vi "Read Recurse.vi"(7 "Append Name (T)":bool=TRUE, 8 "Error In":errorcluster, 9 "Variant DB":variant, 10 "Name":string, 11 "Variant":variant) -> (0 "Error Out":errorcluster, 2 "String":string)   [LabVIEW 2017, in "Configit.lvlib"]
uses:
  Configit.lvlib
  <vilib>/Waveform/DTblOps.llb/DTbl Empty Digital.vi
  <vilib>/Waveform/DWDTOps.llb/DWDT Empty Digital.vi
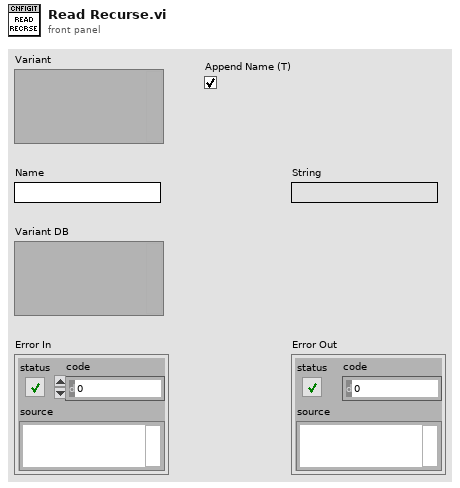
[diagram p1: front panel]
types:
  T1 = typedef "VariantType.lvlib/Type.ctl" = enum8{"Invalid Type", "Void", "I8", "I16", "I32", "I64", "U8", "U16", "U32", "U64", "Single Float", "Double Float", "Extended Float", "Single Complex", "Double Complex", "Extended Complex", "Enum U8", "Enum U16", "Enum U32", "Enum U64", "Single Float With Unit", "Double Float With Unit", "Extended Float With Unit", "Single Complex with Unit", "Double Complex with Unit", "Extended Complex with Unit", "Boolean", "String", "Path", "Picture", "Tag", "Array", "Cluster", "Variant", "LV Variant", "Waveform", "Timestamp", "Digital Waveform", "Digital Data", "ExpressData", "Refnum", "External Data", "VI", "Poly VI", "LabVIEW Class Instance", "Fixed Point"}
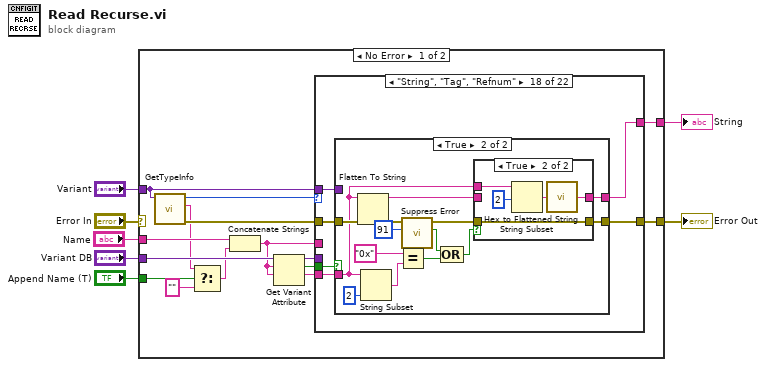
[diagram p0: block diagram]
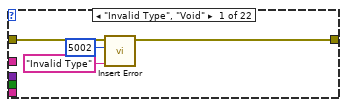
[diagram p2: hidden frame]
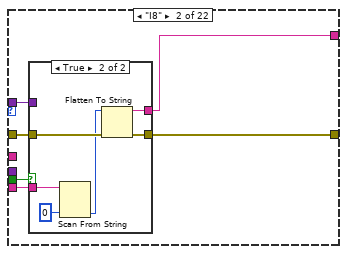
[diagram p3: hidden frame]
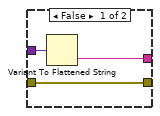
[diagram p4: hidden frame]
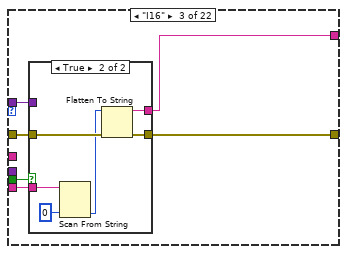
[diagram p5: hidden frame]
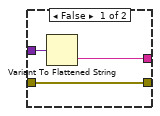
[diagram p6: hidden frame]
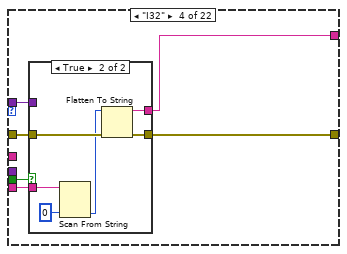
[diagram p7: hidden frame]
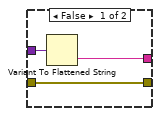
[diagram p8: hidden frame]
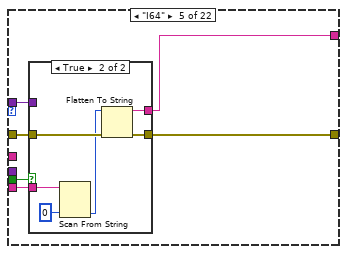
[diagram p9: hidden frame]
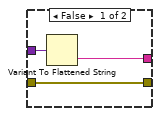
[diagram p10: hidden frame]
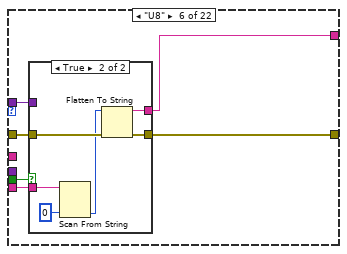
[diagram p11: hidden frame]
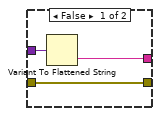
[diagram p12: hidden frame]
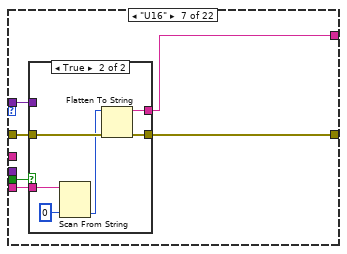
[diagram p13: hidden frame]
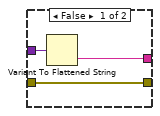
[diagram p14: hidden frame]
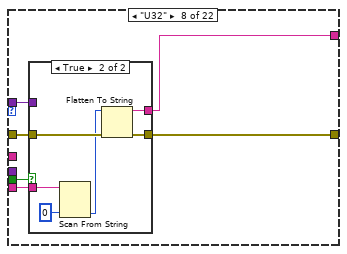
[diagram p15: hidden frame]
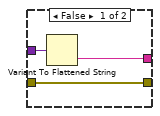
[diagram p16: hidden frame]
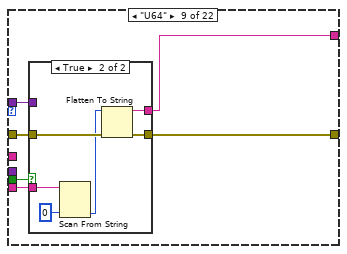
[diagram p17: hidden frame]
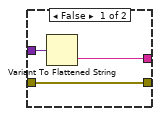
[diagram p18: hidden frame]
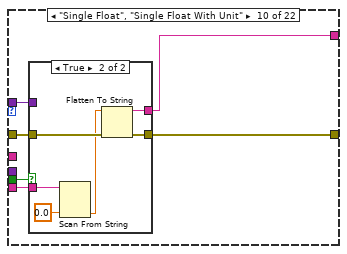
[diagram p19: hidden frame]
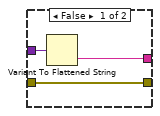
[diagram p20: hidden frame]
diagram:
  n1 = case shown="No Error" "Error In" {
    selector: "Error In" -> [_ w387]
    tunnel: "Variant" -> [w21 _]
    tunnel: "Name" -> [w18 _]
    tunnel: [w19 w387] -> w4
    tunnel: "Variant DB" -> [w17 _]
    tunnel: [w12 _] -> w2
    tunnel: "Append Name (T)" -> [w11 _]
    frame No Error {
      n2 = call "GetTypeInfo.vi"("Variant"=w21) -> ("Error Out"=w20:errorcluster, "Name"=w10:string, "Type Enum"=w22:T1)  [unwired: 7 in, 1 out]
      n3 = Select(t=w10, s=w11, f="") -> (s? t:f=w9:string)
      n4 = Concatenate Strings(w18, w9) -> (w13:string)
      n5 = Get Variant Attribute(Variant=w17, name=w13, default value (empty Variant)=w13) -> (duplicate Variant=w14:variant, found=w16:bool, value=w15:string)  [unwired: 1 in, 1 out]
      n6 = case shown="\"String\", \"Tag\", \"Refnum\"" w22 {
        tunnel: w21 -> [_ w28 w43 w58 w73 w88 w103 w118 w133 w148 w163 w178 w193 w214 w235 w256 w277 w293 w323 w339 w364 w374]
        tunnel: w20 -> [w26 w31 w46 w61 w76 w91 w106 w121 w136 w151 w166 w181 w196 w217 w238 w259 w280 w296 w326 w342 w365 w377]
        tunnel: [w23 w29 w44 w59 w74 w89 w104 w119 w134 w149 w164 w179 w194 w215 w236 w257 w278 w294 w324 w340 w354 w375] -> w19
        tunnel: w16 -> [_ w30 w45 w60 w75 w90 w105 w120 w135 w150 w165 w180 w195 w216 w237 w258 w279 w295 w325 w341 _ w376]
        tunnel: w15 -> [_ w32 w47 w62 w77 w92 w107 w122 w137 w152 w167 w182 w197 w218 w239 w260 w281 w297 w327 w343 _ w378]
        tunnel: w14 -> [_ _ _ _ _ _ _ _ _ _ _ _ _ _ _ _ _ _ _ w337 w362 _]
        tunnel: w13 -> [_ _ _ _ _ _ _ _ _ _ _ _ _ _ _ _ _ _ _ w336 w357 _]
        tunnel: [_ w27 w42 w57 w72 w87 w102 w117 w132 w147 w162 w177 w192 w213 w234 w255 w276 w292 w322 w338 w355 w373] -> w12
        frame "Invalid Type", "Void" {
          n7 = call "Insert Error.vi"("Message"="Invalid Type", "Code (5000)"=5002, "Error In"=w26) -> ("Error Out"=w23:errorcluster)  [unwired: 8 in]
        }
        frame "I8" {
          n8 = case shown="True" w30 {
            tunnel: w32 -> [_ w41]
            tunnel: w31 -> [w35 w40]
            tunnel: [w35 w39] -> w29
            tunnel: [w34 w38] -> w27
            tunnel: w28 -> [w33 _]
            frame False {
              n9 = Variant To Flattened String(Variant=w33) -> (data string=w34:string)  [unwired: 1 out]
            }
            frame True {
              n10 = Scan From String(input string=w41, default 1=i8 0 ("default (0 I32)")) -> (output 1=w37:i8)  [unwired: 3 in, 3 out]
              n11 = Flatten To String(anything=w37, error in (no error)=w40) -> (data string=w38:string, error out=w39:errorcluster)  [unwired: 2 in, 1 out]
            }
          }
        }
        frame "I16" {
          n12 = case shown="True" w45 {
            tunnel: w47 -> [_ w56]
            tunnel: w46 -> [w50 w55]
            tunnel: [w50 w54] -> w44
            tunnel: [w49 w53] -> w42
            tunnel: w43 -> [w48 _]
            frame False {
              n13 = Variant To Flattened String(Variant=w48) -> (data string=w49:string)  [unwired: 1 out]
            }
            frame True {
              n14 = Scan From String(input string=w56, default 1=i16 0 ("default (0 I32)")) -> (output 1=w52:i16)  [unwired: 3 in, 3 out]
              n15 = Flatten To String(anything=w52, error in (no error)=w55) -> (data string=w53:string, error out=w54:errorcluster)  [unwired: 2 in, 1 out]
            }
          }
        }
        frame "I32" {
          n16 = case shown="True" w60 {
            tunnel: w62 -> [_ w71]
            tunnel: w61 -> [w65 w70]
            tunnel: [w65 w69] -> w59
            tunnel: [w64 w68] -> w57
            tunnel: w58 -> [w63 _]
            frame False {
              n17 = Variant To Flattened String(Variant=w63) -> (data string=w64:string)  [unwired: 1 out]
            }
            frame True {
              n18 = Scan From String(input string=w71, default 1=0 ("default (0 I32)")) -> (output 1=w67:i32)  [unwired: 3 in, 3 out]
              n19 = Flatten To String(anything=w67, error in (no error)=w70) -> (data string=w68:string, error out=w69:errorcluster)  [unwired: 2 in, 1 out]
            }
          }
        }
        frame "I64" {
          n20 = case shown="True" w75 {
            tunnel: w77 -> [_ w86]
            tunnel: w76 -> [w80 w85]
            tunnel: [w80 w84] -> w74
            tunnel: [w79 w83] -> w72
            tunnel: w73 -> [w78 _]
            frame False {
              n21 = Variant To Flattened String(Variant=w78) -> (data string=w79:string)  [unwired: 1 out]
            }
            frame True {
              n22 = Scan From String(input string=w86, default 1=i64 0 ("default (0 I32)")) -> (output 1=w82:i64)  [unwired: 3 in, 3 out]
              n23 = Flatten To String(anything=w82, error in (no error)=w85) -> (data string=w83:string, error out=w84:errorcluster)  [unwired: 2 in, 1 out]
            }
          }
        }
        frame "U8" {
          n24 = case shown="True" w90 {
            tunnel: w92 -> [_ w101]
            tunnel: w91 -> [w95 w100]
            tunnel: [w95 w99] -> w89
            tunnel: [w94 w98] -> w87
            tunnel: w88 -> [w93 _]
            frame False {
              n25 = Variant To Flattened String(Variant=w93) -> (data string=w94:string)  [unwired: 1 out]
            }
            frame True {
              n26 = Scan From String(input string=w101, default 1=u8 0 ("default (0 I32)")) -> (output 1=w97:u8)  [unwired: 3 in, 3 out]
              n27 = Flatten To String(anything=w97, error in (no error)=w100) -> (data string=w98:string, error out=w99:errorcluster)  [unwired: 2 in, 1 out]
            }
          }
        }
        frame "U16" {
          n28 = case shown="True" w105 {
            tunnel: w107 -> [_ w116]
            tunnel: w106 -> [w110 w115]
            tunnel: [w110 w114] -> w104
            tunnel: [w109 w113] -> w102
            tunnel: w103 -> [w108 _]
            frame False {
              n29 = Variant To Flattened String(Variant=w108) -> (data string=w109:string)  [unwired: 1 out]
            }
            frame True {
              n30 = Scan From String(input string=w116, default 1=u16 0 ("default (0 I32)")) -> (output 1=w112:u16)  [unwired: 3 in, 3 out]
              n31 = Flatten To String(anything=w112, error in (no error)=w115) -> (data string=w113:string, error out=w114:errorcluster)  [unwired: 2 in, 1 out]
            }
          }
        }
        frame "U32" {
          n32 = case shown="True" w120 {
            tunnel: w122 -> [_ w131]
            tunnel: w121 -> [w125 w130]
            tunnel: [w125 w129] -> w119
            tunnel: [w124 w128] -> w117
            tunnel: w118 -> [w123 _]
            frame False {
              n33 = Variant To Flattened String(Variant=w123) -> (data string=w124:string)  [unwired: 1 out]
            }
            frame True {
              n34 = Scan From String(input string=w131, default 1=u32 0 ("default (0 I32)")) -> (output 1=w127:u32)  [unwired: 3 in, 3 out]
              n35 = Flatten To String(anything=w127, error in (no error)=w130) -> (data string=w128:string, error out=w129:errorcluster)  [unwired: 2 in, 1 out]
            }
          }
        }
        frame "U64" {
          n36 = case shown="True" w135 {
            tunnel: w137 -> [_ w146]
            tunnel: w136 -> [w140 w145]
            tunnel: [w140 w144] -> w134
            tunnel: [w139 w143] -> w132
            tunnel: w133 -> [w138 _]
            frame False {
              n37 = Variant To Flattened String(Variant=w138) -> (data string=w139:string)  [unwired: 1 out]
            }
            frame True {
              n38 = Scan From String(input string=w146, default 1=u64 0 ("default (0 I32)")) -> (output 1=w142:u64)  [unwired: 3 in, 3 out]
              n39 = Flatten To String(anything=w142, error in (no error)=w145) -> (data string=w143:string, error out=w144:errorcluster)  [unwired: 2 in, 1 out]
            }
          }
        }
        frame "Single Float", "Single Float With Unit" {
          n40 = case shown="True" w150 {
            tunnel: w152 -> [_ w161]
            tunnel: w151 -> [w155 w160]
            tunnel: [w155 w159] -> w149
            tunnel: [w154 w158] -> w147
            tunnel: w148 -> [w153 _]
            frame False {
              n41 = Variant To Flattened String(Variant=w153) -> (data string=w154:string)  [unwired: 1 out]
            }
            frame True {
              n42 = Scan From String(input string=w161, default 1=sgl 0.0 ("default (0 I32)")) -> (output 1=w157:sgl)  [unwired: 3 in, 3 out]
              n43 = Flatten To String(anything=w157, error in (no error)=w160) -> (data string=w158:string, error out=w159:errorcluster)  [unwired: 2 in, 1 out]
            }
          }
        }
        frame "Double Float", "Double Float With Unit" {
          n44 = case shown="True" w165 {
            tunnel: w167 -> [_ w176]
            tunnel: w166 -> [w170 w175]
            tunnel: [w170 w174] -> w164
            tunnel: [w169 w173] -> w162
            tunnel: w163 -> [w168 _]
            frame False {
              n45 = Variant To Flattened String(Variant=w168) -> (data string=w169:string)  [unwired: 1 out]
            }
            frame True {
              n46 = Scan From String(input string=w176, default 1=0.0 ("default (0 I32)")) -> (output 1=w172:dbl)  [unwired: 3 in, 3 out]
              n47 = Flatten To String(anything=w172, error in (no error)=w175) -> (data string=w173:string, error out=w174:errorcluster)  [unwired: 2 in, 1 out]
            }
          }
        }
        frame "Extended Float", "Extended Float With Unit" {
          n48 = case shown="True" w180 {
            tunnel: w182 -> [_ w191]
            tunnel: w181 -> [w185 w190]
            tunnel: [w185 w189] -> w179
            tunnel: [w184 w188] -> w177
            tunnel: w178 -> [w183 _]
            frame False {
              n49 = Variant To Flattened String(Variant=w183) -> (data string=w184:string)  [unwired: 1 out]
            }
            frame True {
              n50 = Scan From String(input string=w191, default 1=ext 0.0 ("default (0 I32)")) -> (output 1=w187:ext)  [unwired: 3 in, 3 out]
              n51 = Flatten To String(anything=w187, error in (no error)=w190) -> (data string=w188:string, error out=w189:errorcluster)  [unwired: 2 in, 1 out]
            }
          }
        }
        frame "Enum U8" {
          n52 = case shown="True" w195 {
            tunnel: w197 -> [_ w207]
            tunnel: w196 -> [w200 w201]
            tunnel: [w200 w212] -> w194
            tunnel: [w199 w211] -> w192
            tunnel: w193 -> [w198 w210]
            frame False {
              n53 = Variant To Flattened String(Variant=w198) -> (data string=w199:string)  [unwired: 1 out]
            }
            frame True {
              n54 = dll-call lib="LabVIEW" fn="GVariantTDR_GetEnumInfo"("lvVar"=w210, string[] []) -> (w208:string[])  [unwired: 5 in, 2 out]
              n55 = Search 1D Array(1D array=w208, element=w207) -> (index of element=w203:i32)  [unwired: 1 in]
              n56 = In Range and Coerce(upper limit=255, x=w203, lower limit=0) -> (coerced(x)=w202:i32)  [unwired: 1 out]
              n57 = To Unsigned Byte Integer(number=w202) -> (unsigned 8bit integer=w206:u8)
              n58 = Flatten To String(anything=w206, error in (no error)=w201) -> (data string=w211:string, error out=w212:errorcluster)  [unwired: 2 in, 1 out]
            }
          }
        }
        frame "Enum U16" {
          n59 = case shown="True" w216 {
            tunnel: w218 -> [_ w228]
            tunnel: w217 -> [w221 w222]
            tunnel: [w221 w233] -> w215
            tunnel: [w220 w232] -> w213
            tunnel: w214 -> [w219 w231]
            frame False {
              n60 = Variant To Flattened String(Variant=w219) -> (data string=w220:string)  [unwired: 1 out]
            }
            frame True {
              n61 = dll-call lib="LabVIEW" fn="GVariantTDR_GetEnumInfo"("lvVar"=w231, string[] []) -> (w229:string[])  [unwired: 5 in, 2 out]
              n62 = Search 1D Array(1D array=w229, element=w228) -> (index of element=w224:i32)  [unwired: 1 in]
              n63 = In Range and Coerce(upper limit=65535, x=w224, lower limit=0) -> (coerced(x)=w223:i32)  [unwired: 1 out]
              n64 = To Unsigned Word Integer(number=w223) -> (unsigned 16bit integer=w227:u16)
              n65 = Flatten To String(anything=w227, error in (no error)=w222) -> (data string=w232:string, error out=w233:errorcluster)  [unwired: 2 in, 1 out]
            }
          }
        }
        frame "Enum U32" {
          n66 = case shown="True" w237 {
            tunnel: w239 -> [_ w249]
            tunnel: w238 -> [w242 w243]
            tunnel: [w242 w254] -> w236
            tunnel: [w241 w253] -> w234
            tunnel: w235 -> [w240 w252]
            frame False {
              n67 = Variant To Flattened String(Variant=w240) -> (data string=w241:string)  [unwired: 1 out]
            }
            frame True {
              n68 = dll-call lib="LabVIEW" fn="GVariantTDR_GetEnumInfo"("lvVar"=w252, string[] []) -> (w250:string[])  [unwired: 5 in, 2 out]
              n69 = Search 1D Array(1D array=w250, element=w249) -> (index of element=w245:i32)  [unwired: 1 in]
              n70 = In Range and Coerce(upper limit=2147483647, x=w245, lower limit=0) -> (coerced(x)=w244:i32)  [unwired: 1 out]
              n71 = To Unsigned Long Integer(number=w244) -> (unsigned 32bit integer=w248:u32)
              n72 = Flatten To String(anything=w248, error in (no error)=w243) -> (data string=w253:string, error out=w254:errorcluster)  [unwired: 2 in, 1 out]
            }
          }
        }
        frame "Enum U64" {
          n73 = case shown="True" w258 {
            tunnel: w260 -> [_ w270]
            tunnel: w259 -> [w263 w264]
            tunnel: [w263 w275] -> w257
            tunnel: [w262 w274] -> w255
            tunnel: w256 -> [w261 w273]
            frame False {
              n74 = Variant To Flattened String(Variant=w261) -> (data string=w262:string)  [unwired: 1 out]
            }
            frame True {
              n75 = dll-call lib="LabVIEW" fn="GVariantTDR_GetEnumInfo"("lvVar"=w273, string[] []) -> (w271:string[])  [unwired: 5 in, 2 out]
              n76 = Search 1D Array(1D array=w271, element=w270) -> (index of element=w266:i32)  [unwired: 1 in]
              n77 = In Range and Coerce(upper limit=2147483647, x=w266, lower limit=0) -> (coerced(x)=w265:i32)  [unwired: 1 out]
              n78 = To Unsigned Quad Integer(1:w265) -> (0:w269:u64)
              n79 = Flatten To String(anything=w269, error in (no error)=w264) -> (data string=w274:string, error out=w275:errorcluster)  [unwired: 2 in, 1 out]
            }
          }
        }
        frame "Boolean" {
          n80 = case shown="True" w279 {
            tunnel: w281 -> [_ w285]
            tunnel: w280 -> [w284 w290]
            tunnel: [w284 w289] -> w278
            tunnel: [w283 w288] -> w276
            tunnel: w277 -> [w282 _]
            frame False {
              n81 = Variant To Flattened String(Variant=w282) -> (data string=w283:string)  [unwired: 1 out]
            }
            frame True {
              n82 = To Lower Case(string=w285) -> (all lower case string=w287:string)
              n83 = case shown="\"1\", \"on\", \"true\", \"yes\"" w287 {
                tunnel: [_ TRUE] -> w286
                frame Default {
                }
                frame "1", "on", "true", "yes" {
                }
              }
              n84 = Flatten To String(anything=w286, error in (no error)=w290) -> (data string=w288:string, error out=w289:errorcluster)  [unwired: 2 in, 1 out]
            }
          }
        }
        frame "String", "Tag", "Refnum" {
          n85 = case shown="True" w295 {
            tunnel: w297 -> [_ w306]
            tunnel: w296 -> [w300 w314]
            tunnel: [w300 w310] -> w294
            tunnel: [w299 w309] -> w292
            tunnel: w293 -> [w298 _]
            frame False {
              n86 = Variant To Flattened String(Variant=w298) -> (data string=w299:string)  [unwired: 1 out]
            }
            frame True {
              n87 = Flatten To String(anything=w306, error in (no error)=w314) -> (data string=w311:string, error out=w312:errorcluster)  [unwired: 2 in, 1 out]
              n88 = String Subset(string=w306, length (rest)=2 ("length (rest)")) -> (substring=w304:string)  [unwired: 1 in]
              n89 = Equal?(x="0x" ("y"), y=w304) -> (x = y?=w303:bool)
              n90 = call "Suppress Error.vi"("Error Code"=91, "Error In"=w312) -> ("Error Supressed?"=w302:bool, "Error Out"=w308:errorcluster)  [unwired: 4 in]
              n91 = Compound Arithmetic op=OR(w302, w303) -> (w301:bool)
              n92 = case shown="True" w301 {
                tunnel: [w316 w317] -> w309
                tunnel: w311 -> [w316 _]
                tunnel: w308 -> [w315 w321]
                tunnel: [w315 w321] -> w310
                tunnel: w306 -> [_ w318]
                frame False {
                }
                frame True {
                  n93 = String Subset(string=w318, offset (0)=2) -> (substring=w319:string)  [unwired: 1 in]
                  n94 = call "Hex to Flattened String.vi"("Hex"=w319) -> ("Flattened String"=w317:string)
                }
              }
            }
          }
        }
        frame "Path" {
          n95 = case shown="True" w325 {
            tunnel: w327 -> [_ w332]
            tunnel: w326 -> [w330 w335]
            tunnel: [w330 w334] -> w324
            tunnel: [w329 w333] -> w322
            tunnel: w323 -> [w328 _]
            frame False {
              n96 = Variant To Flattened String(Variant=w328) -> (data string=w329:string)  [unwired: 1 out]
            }
            frame True {
              n97 = String To Path(string=w332) -> (path=w331:path)
              n98 = Flatten To String(anything=w331, error in (no error)=w335) -> (data string=w333:string, error out=w334:errorcluster)  [unwired: 2 in, 1 out]
            }
          }
        }
        frame "Array" {
          n99 = case shown="True" w341 {
            tunnel: w343 -> [_ w347]
            tunnel: w342 -> [w346 w353]
            tunnel: [w346 w351] -> w340
            tunnel: [w345 w350] -> w338
            tunnel: w339 -> [w344 w352]
            tunnel: w337 -> [_ w349]
            tunnel: w336 -> [_ w348]
            frame False {
              n100 = Variant To Flattened String(Variant=w344) -> (data string=w345:string)  [unwired: 1 out]
            }
            frame True {
              n101 = call "Read Array.vi"("Value"=w347, "Error In"=w353, "Variant DB"=w349, "Name"=w348, "Variant"=w352) -> ("Error Out"=w351:errorcluster, "String"=w350:string)  [unwired: 5 in]
            }
          }
        }
        frame "Cluster" {
          n102 = Variant To Data(error in=w365, type=variant[] [], Variant=w364) -> (data=w361:variant[], error out=w363:errorcluster)
          n103 = Concatenate Strings(w357, "." ("string")) -> (w359:string)
          n104 = for {
            tunnel: w362 -> [w368]
            tunnel: w361 -> [w370] mode=indexing
            tunnel: w359 -> [w367]
            tunnel: [w369] -> w356 mode=indexing
            workers-P: _ -> [_]
            tunnel: w363 -> [w371]
            tunnel: [w372] -> w360 mode=indexing
            n105 = call "Read Recurse.vi"("Error In"=w371, "Variant DB"=w368, "Name"=w367, "Variant"=w370) -> ("Error Out"=w372:errorcluster, "String"=w369:string)  [unwired: 6 in]
          }
          n106 = Concatenate Strings(w356) -> (w355:string)
          n107 = Merge Errors(w360) -> (w354:errorcluster)
        }
        frame Default {
          n108 = case shown="True" w376 {
            tunnel: w378 -> [_ w384]
            tunnel: w377 -> [w381 w386]
            tunnel: [w381 w386] -> w375
            tunnel: [w380 w382] -> w373
            tunnel: w374 -> [w379 _]
            frame False {
              n109 = Variant To Flattened String(Variant=w379) -> (data string=w380:string)  [unwired: 1 out]
            }
            frame True {
              n110 = String Subset(string=w384, offset (0)=2) -> (substring=w383:string)  [unwired: 1 in]
              n111 = call "Hex to Flattened String.vi"("Hex"=w383) -> ("Flattened String"=w382:string)
            }
          }
        }
      }
    }
    frame Error {
    }
  }
  "Error Out" <- w4
  "String" <- w2
